vi "setpoint.vi"(8 "error in (no error)":errorcluster, 11 "Input":string="34,45,89") -> (0 "error out":errorcluster, 3 "Output":string)   [LabVIEW 2014]
uses:
  <userlib>/Nanonis Prog Interface V5/Nanonis Prog Interface.lvlib
panel:
  in  "milliseconds to wait":u32
  out "size(s)":i32=3
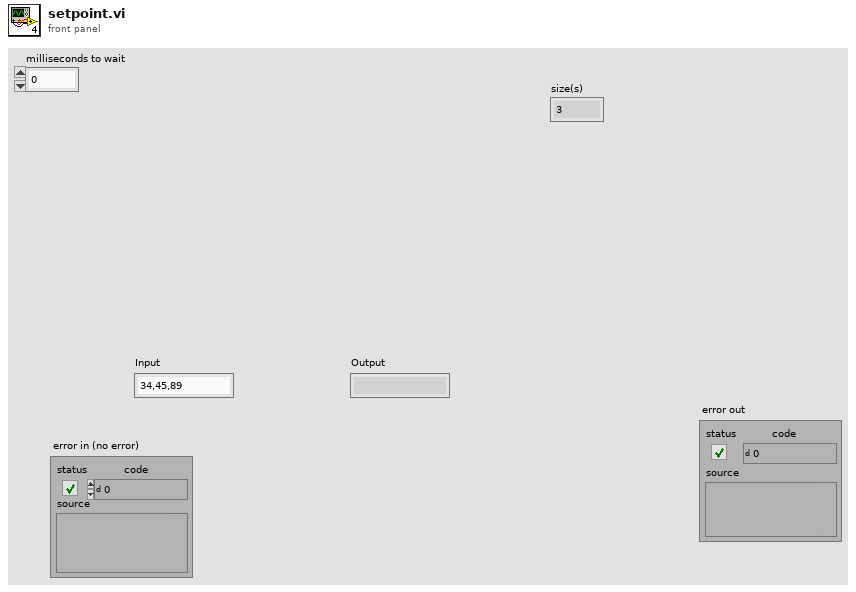
[diagram p1: front panel]
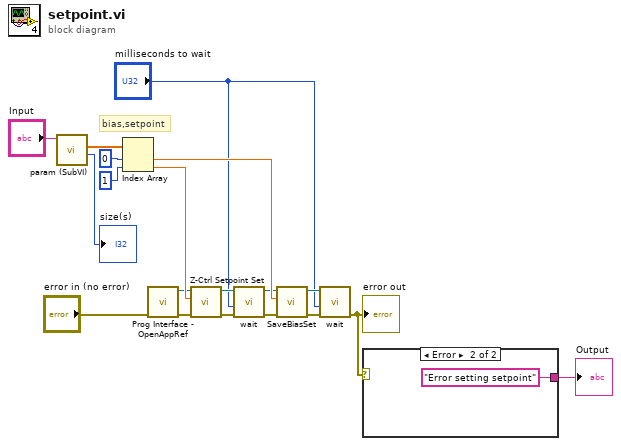
[diagram p0: block diagram]
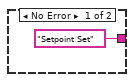
[diagram p2: hidden frame]
diagram:
  # "bias,setpoint"
  n1 = call <userlib>:"param (SubVI).vi"("Input"="Input") -> ("num"=→"size(s)":i32, "parm"=w17:dbl[])  [unwired: 8 in, 1 out]
  n2 = Index Array(array=w17, index #1=0 ("index"), index #2=1 ("index")) -> (element #1=w14:dbl, element #2=w13:dbl)
  n3 = call <userlib>:"Prog Interface - OpenAppRef.vi"("Error in (no error)"="error in (no error)") -> ("Error out"=w5:errorcluster, "Application reference"=w4:refnum<vi>)  [unwired: 5 in]
  n4 = call <userlib>:"Z-Ctrl Setpoint Set.vi"("error in (no error)"=w5, "Z Controller setpoint"=w13, "Application ref in"=w4) -> ("error out"=w9:errorcluster, "Application ref out"=w12:refnum<vi>)  [unwired: 7 in]
  n5 = call "wait.vi"("error in"=w9, "milliseconds to wait"="milliseconds to wait", "application reference in"=w12) -> ("error out"=w10:errorcluster, "application reference out"=w11:refnum<vi>)  [unwired: 7 in]
  n6 = call "SaveBiasSet.vi"("Application ref in"=w11, "Bias (V)"=w14, "error in (no error)"=w10) -> ("Application ref out"=w8:refnum<vi>, "Error out"=w7:errorcluster)  [unwired: 6 in]
  n7 = call "wait.vi"("error in"=w7, "milliseconds to wait"="milliseconds to wait", "application reference in"=w8) -> ("error out"=w2:errorcluster)  [unwired: 7 in, 1 out]
  "error out" <- w2
  n8 = case shown="Error" w2 {
    tunnel: ["Setpoint Set" "Error setting setpoint"] -> w1
    frame No Error {
    }
    frame Error {
    }
  }
  "Output" <- w1
